vi "Destroy User Event - Stop.vi"(8 "error in (no error)":errorcluster, 11 "User events":T1) -> (0 "error out":errorcluster)   [LabVIEW 2020, in "User Event - Stop.lvlib"]
doc: "Destroy the user event, even if there is an incoming error."
uses:
  User Event - Stop.lvlib
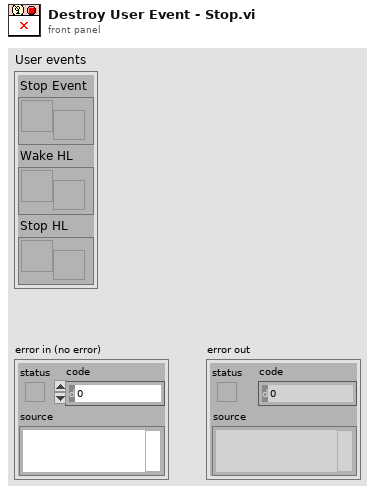
[diagram p1: front panel]
types:
  T1 = cluster{"Stop Event":refnum<user-event>, "Wake HL":refnum<user-event>, "Stop HL":refnum<user-event>}
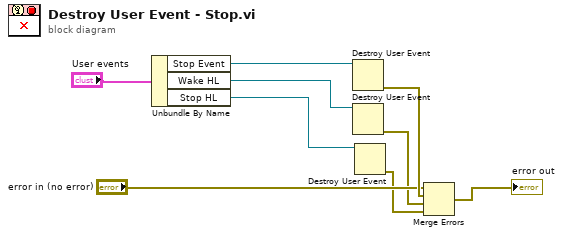
[diagram p0: block diagram]
diagram:
  n1 = Unbundle By Name("User events") -> ("Stop Event"=w6:refnum<user-event>, "Wake HL"=w5:refnum<user-event>, "Stop HL"=w3:refnum<user-event>)
  n2 = Destroy User Event(user event=w6) -> (error out=w9:errorcluster)  [unwired: 1 in]
  n3 = Destroy User Event(user event=w5) -> (error out=w4:errorcluster)  [unwired: 1 in]
  n4 = Destroy User Event(user event=w3) -> (error out=w2:errorcluster)  [unwired: 1 in]
  n5 = Merge Errors("error in (no error)", w9, w4, w2) -> (→"error out":errorcluster)
